vi "BRig_RT_panel_ExpStruct_v1,11.vi"(7 "input_setValues":bool, 11 "input_dataExp":u16[](array[numeric])) -> (3 "output_dataExp":u16[](array[numeric]))   [LabVIEW 2014]
panel:
  in  "I_L_nTrig_PerState":bool
  in  "I_Cue2":bool
  in  "T_Cue2_LED_max":u16=1000 caption="Max" min=5 max=5000 step=5
  in  "T_Cue2_LED_min":u16=1000 caption="Min" min=5 max=5000 step=5
  in  "T_Cue2_LED_step":u16=1000 caption="Penalty" min=1 max=10000 step=1
  in  "T_Cue2_Audio_max":u16=1000 caption="Max" min=5 max=5000 step=5
  in  "T_Cue2_Audio_min":u16=1000 caption="Min" min=5 max=5000 step=5
  in  "T_Cue2_Audio_step":u16=1000 caption="Penalty" min=1 max=10000 step=1
  in  "T_ENL2_step":u16=100 caption="Penalty" min=10 max=10000 step=10
  in  "T_ENL2_max":u16=1000 caption="Max" min=250 max=10000 step=250
  in  "T_ENL2_min":u16=1000 caption="Min" min=250 max=10000 step=250
  in  "ClosedLoop_LaserHold_l2":bool
  in  "ClosedLoop_LaserHold_l1":bool
  in  "FreeReward_Count2":u16
  in  "FreeReward_Count1":u16
  in  "FreeReward_Switch":bool
  in  "T_CuePenalty":u16=1000 caption="Penalty" min=1 max=10000 step=1
  in  "T_ENLPenalty":u16=100 caption="Penalty" min=10 max=10000 step=10
  in  "LaserSwitch_Probability_L1":u16
  in  "LaserSwitch":u16(slide) max=3 step=1 scale=0.0..3.0
  in  "I_allReward":bool caption="NonSpecific\nLick Direction"
  in  "Tcycle_Reward_max_R":u16=1000 caption="Max" min=5 max=5000 step=5
  in  "Tcycle_Reward_min_R":u16=1000 caption="Min" min=5 max=5000 step=5
  in  "Tcycle_Reward_step_R":u16=1000 caption="Penalty" min=1 max=10000 step=1
  in  "Tcycle_Reward_max_L":u16=1000 caption="Max" min=5 max=5000 step=5
  in  "Tcycle_Reward_min_L":u16=1000 caption="Min" min=5 max=5000 step=5
  in  "Tcycle_Reward_step_L":u16=1000 caption="Penalty" min=1 max=10000 step=1
  in  "T_Cue_LED_max":u16=1000 caption="Max" min=5 max=5000 step=5
  in  "T_Cue_LED_min":u16=1000 caption="Min" min=5 max=5000 step=5
  in  "T_Cue_LED_step":u16=1000 caption="Penalty" min=1 max=10000 step=1
  in  "SolenoidProbability_L":u16=100 caption="Reward Time [ms]" min=1 max=1000 step=1
  in  "SolenoidProbability_R":u16=100 caption="Reward Time [ms]" min=1 max=1000 step=1
  in  "T_Cue_Audio_max":u16=1000 caption="Max" min=5 max=5000 step=5
  in  "T_Cue_Audio_min":u16=1000 caption="Min" min=5 max=5000 step=5
  in  "BUR_max":u16 caption="Count Reward Structure  (0 = off)"
  in  "Tcycle_Timeout":u16=1000 caption="Timeout Time [ms]" min=10 max=10000 step=1
  in  "Tcycle_Wrong":u16=1000 caption="Wrong Time [ms]" min=10 max=10000 step=1
  in  "Tcycle_Selection":u16=1000 caption="Answer Time [ms]" min=1 max=10000 step=1
  in  "Tcycle_RewardPost":u16=1000 caption="Consumption Time [ms]" min=250 max=10000 step=250
  in  "TpB_Max_R":u16=4 caption="Max TrialsPerBlock" min=1 max=12 step=1
  in  "TpB_Min_R":u16=4 caption="Min TrialsPerBlock" min=1 max=12 step=1
  in  "TpB_Max_L":u16=4 caption="Max TrialsPerBlock" min=1 max=12 step=1
  in  "TpB_Min_L":u16=4 caption="Min TrialsPerBlock" min=1 max=12 step=1
  in  "BUR_min":u16 caption="Count Reward Structure\n(0 = off)"
  in  "TrialUntilReward":bool caption="Ignore Wrong\nSelection"
  in  "T_Cue_Audio_step":u16=1000 caption="Penalty" min=1 max=10000 step=1
  in  "T_ENL_step":u16=100 caption="Penalty" min=10 max=10000 step=10
  in  "T_ENL_max":u16=1000 caption="Max" min=250 max=10000 step=250
  in  "T_ENL_min":u16=1000 caption="Min" min=250 max=10000 step=250
  # "Experiment Task Structure"
  # "Min            Max               Step        Penalty"
  # "(Laser1 or Laser2)\nLaser1 probability"
  # "Enforced\nNonLick"
  # "Cue Audio"
  # "(ClosedLoop Structure)"
  # "Hold Laser1"
  # "Hold Laser2"
  # "Cue LED"
  # "Allow Multiple Laser\nTriggers During\nENL and Cue?"
  # "Min            Max               Step"
  # "ENL 2"
  # "Cue 2 Audio"
  # "Cue 2 LED"
  # "Selection"
  # "Min"
  # "Max"
  # "Reward - Dispense Water"
  # "Min            Max            StepSize"
  # "Left"
  # "Trial Per Block Structure \n               Left                        Right"
  # "Right"
  # "Min"
  # "Dispense Water Probability"
  # "Max"
  # "%"
  # "Left"
  # "Right"
  # "%"
  # "Give Reward\nIf Too Many Errors"
  # "Reward - Consumption"
  # "# consecutive ReBiasing trials"
  # "Penalty - Wrong Choice"
  # "# consecutive NonForcedError trials"
  # "Penalty - Choice Timeout"
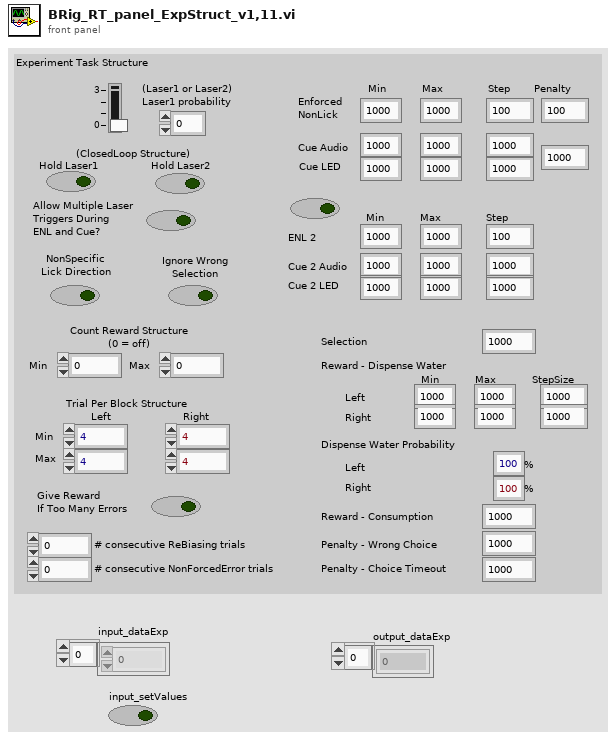
[diagram p1: front panel]
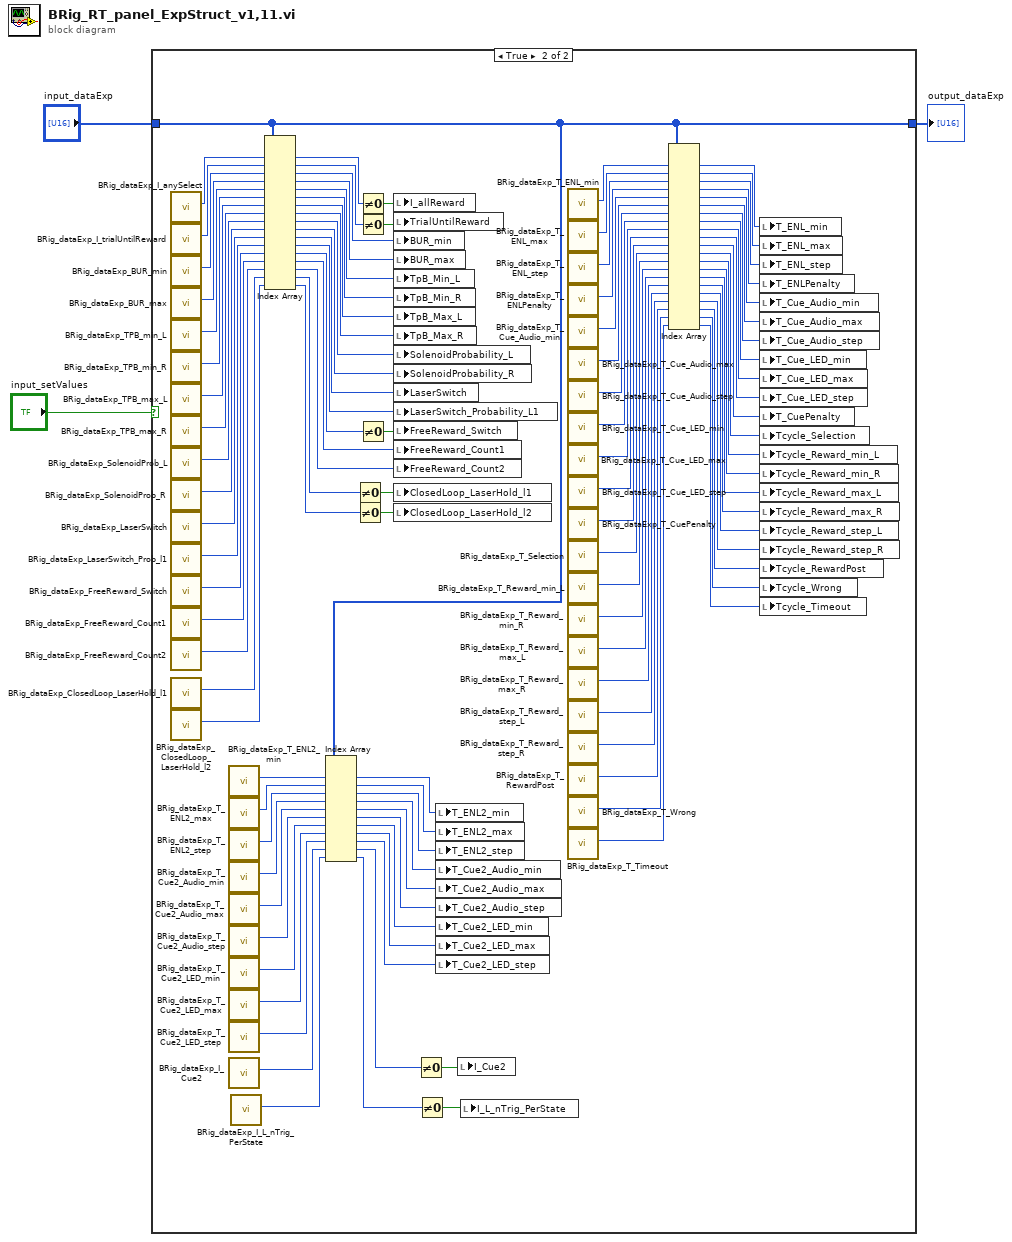
[diagram p0: block diagram]
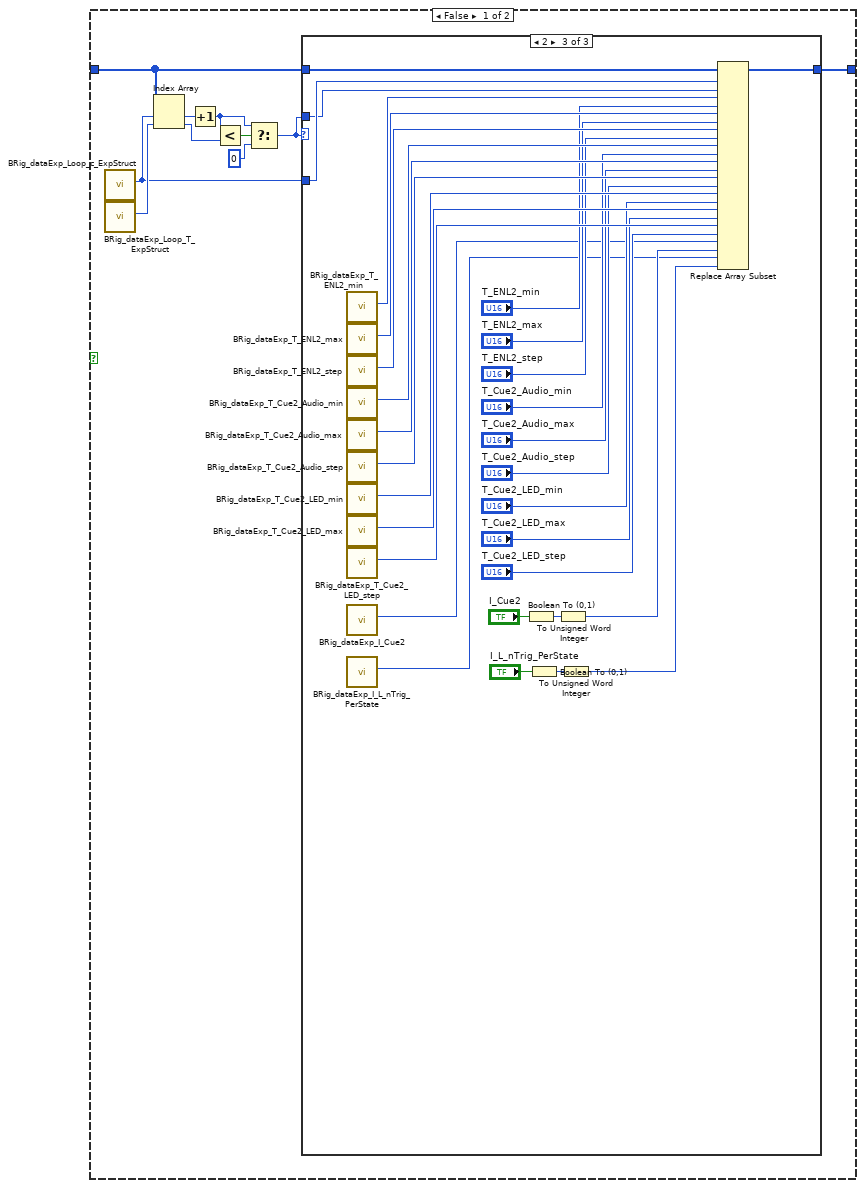
[diagram p2: hidden frame]
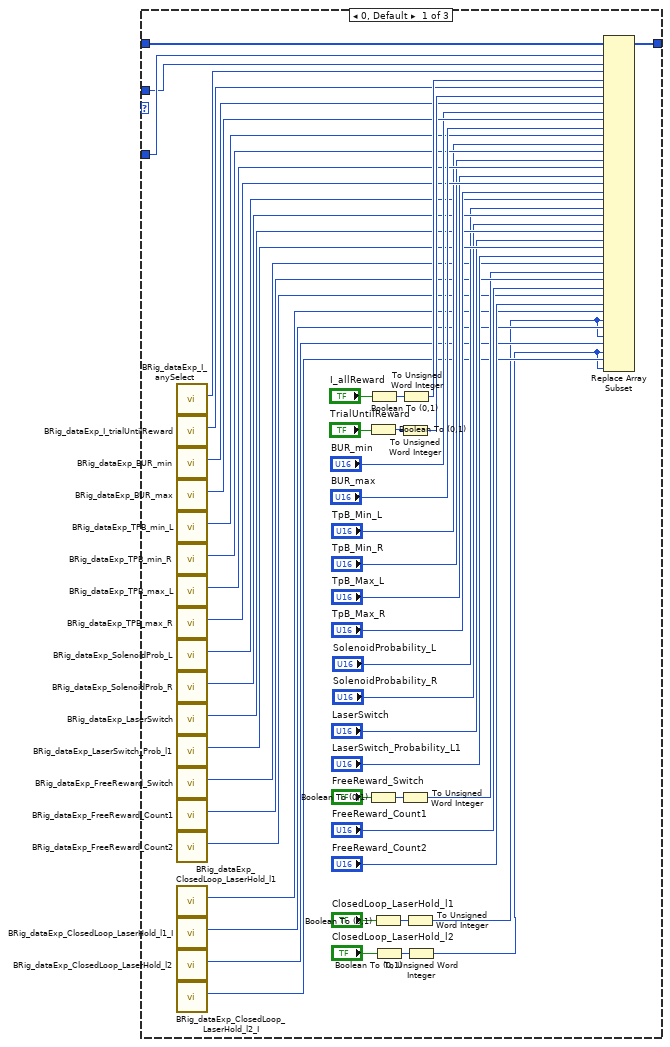
[diagram p3: hidden frame]
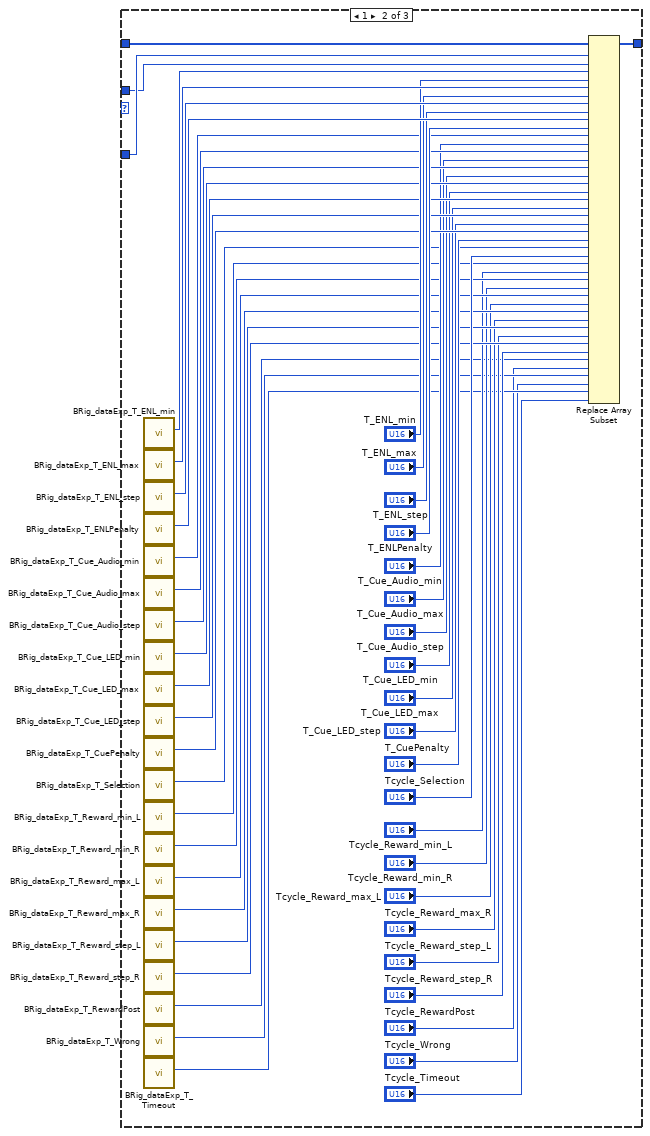
[diagram p4: hidden frame]
diagram:
  n1 = case shown="True" "input_setValues" {
    tunnel: [w13 w164] -> w3
    tunnel: "input_dataExp" -> [w12 w164]
    frame False {
      n2 = call "BRig_dataExp_Loop_c_ExpStruct.vi"() -> ("output_Loop_c_ExpStruct"=w6:i32)  [unwired: 11 in]
      n3 = call "BRig_dataExp_Loop_T_ExpStruct.vi"() -> ("output_Loop_T_ExpStruct"=w11:i32)  [unwired: 11 in]
      n4 = Index Array(array=w12, index #1=w6, index #2=w11) -> (element #1=w10:u16, element #2=w9:u16)
      n5 = Increment(x=w10) -> (x+1=w5:u16)
      n6 = Less?(x=w5, y=w9) -> (x < y?=w8:bool)
      n7 = Select(t=w5, s=w8, f=u16 0) -> (s? t:f=w4:u16)
      n8 = case shown="2" w4 {
        tunnel: w12 -> [w63 w109 w139]
        tunnel: [w62 w108 w138] -> w13
        tunnel: w6 -> [w33 w107 w137]
        tunnel: w4 -> [w32 w106 w136]
        frame 0, Default {
          n9 = call "BRig_dataExp_I_anySelect.vi"() -> ("output_I_anySelect"=w61:i32)  [unwired: 11 in]
          n10 = call "BRig_dataExp_I_trialUntilReward.vi"() -> ("output_I_trialUntilReward"=w57:i32)  [unwired: 11 in]
          n11 = call "BRig_dataExp_BUR_min.vi"() -> ("output_BUR_min"=w53:i32)  [unwired: 11 in]
          n12 = call "BRig_dataExp_BUR_max.vi"() -> ("output_BUR_max"=w52:i32)  [unwired: 11 in]
          n13 = call "BRig_dataExp_TPB_min_L.vi"() -> ("output_TPB_min_L"=w49:i32)  [unwired: 11 in]
          n14 = call "BRig_dataExp_TPB_min_R.vi"() -> ("output_TPB_min_R"=w48:i32)  [unwired: 11 in]
          n15 = call "BRig_dataExp_TPB_max_L.vi"() -> ("output_TPB_max_L"=w47:i32)  [unwired: 11 in]
          n16 = call "BRig_dataExp_TPB_max_R.vi"() -> ("output_TPB_max_R"=w46:i32)  [unwired: 11 in]
          n17 = call "BRig_dataExp_SolenoidProb_L.vi"() -> ("output_SolenoidProbability_L"=w41:i32)  [unwired: 11 in]
          n18 = call "BRig_dataExp_SolenoidProb_R.vi"() -> ("output_SolenoidProbability_R"=w40:i32)  [unwired: 11 in]
          n19 = call "BRig_dataExp_LaserSwitch.vi"() -> ("output_LaserSwitch"=w39:i32)  [unwired: 11 in]
          n20 = call "BRig_dataExp_LaserSwitch_Prob_l1.vi"() -> ("output_LaserSwitch_Probability_L1"=w38:i32)  [unwired: 11 in]
          n21 = call "BRig_dataExp_FreeReward_Switch.vi"() -> ("output_FreeReward_Switch"=w29:i32)  [unwired: 11 in]
          n22 = call "BRig_dataExp_FreeReward_Count1.vi"() -> ("output_FreeReward_Count"=w28:i32)  [unwired: 11 in]
          n23 = call "BRig_dataExp_FreeReward_Count2.vi"() -> ("output_FreeReward_Count"=w25:i32)  [unwired: 11 in]
          n24 = call "BRig_dataExp_ClosedLoop_LaserHold_l1.vi"() -> ("output_CloseLoop_LaserHold_l1"=w23:i32)  [unwired: 11 in]
          n25 = call "BRig_dataExp_ClosedLoop_LaserHold_l1_I.vi"() -> ("output_CloseLoop_LaserHold_l1_I"=w22:i32)  [unwired: 11 in]
          n26 = call "BRig_dataExp_ClosedLoop_LaserHold_l2.vi"() -> ("output_CloseLoop_LaserHold_l2"=w21:i32)  [unwired: 11 in]
          n27 = call "BRig_dataExp_ClosedLoop_LaserHold_l2_I.vi"() -> ("output_CloseLoop_LaserHold_l2_I"=w20:i32)  [unwired: 11 in]
          n28 = Boolean To (0,1)(Boolean="TrialUntilReward") -> (0, 1=w56:i16)
          n29 = Boolean To (0,1)(Boolean="FreeReward_Switch") -> (0, 1=w31:i16)
          n30 = Boolean To (0,1)(Boolean="I_allReward") -> (0, 1=w59:i16)
          n31 = Boolean To (0,1)(Boolean="ClosedLoop_LaserHold_l1") -> (0, 1=w19:i16)
          n32 = Boolean To (0,1)(Boolean="ClosedLoop_LaserHold_l2") -> (0, 1=w17:i16)
          n33 = To Unsigned Word Integer(number=w56) -> (unsigned 16bit integer=w54:u16)
          n34 = To Unsigned Word Integer(number=w31) -> (unsigned 16bit integer=w27:u16)
          n35 = To Unsigned Word Integer(number=w59) -> (unsigned 16bit integer=w58:u16)
          n36 = To Unsigned Word Integer(number=w19) -> (unsigned 16bit integer=w15:u16)
          n37 = To Unsigned Word Integer(number=w17) -> (unsigned 16bit integer=w14:u16)
          n38 = Replace Array Subset(array=w63, new element #1=w32, index #1=w33, new element #2=w58, index #2=w61, new element #3=w54, index #3=w57, new element #4="BUR_min", index #4=w53, new element #5="BUR_max", index #5=w52, new element #6="TpB_Min_L", index #6=w49, new element #7="TpB_Min_R", index #7=w48, new element #8="TpB_Max_L", index #8=w47, new element #9="TpB_Max_R", index #9=w46, new element #10="SolenoidProbability_L", index #10=w41, new element #11="SolenoidProbability_R", index #11=w40, new element #12="LaserSwitch", index #12=w39, new element #13="LaserSwitch_Probability_L1", index #13=w38, new element #14=w27, index #14=w29, new element #15="FreeReward_Count1", index #15=w28, new element #16="FreeReward_Count2", index #16=w25, new element #17=w15, index #17=w23, new element #18=w15, index #18=w22, new element #19=w14, index #19=w21, new element #20=w14, index #20=w20) -> (w62:u16[])
        }
        frame 1 {
          n39 = call "BRig_dataExp_T_ENL_min.vi"() -> ("output_T_ENL_min"=w105:i32)  [unwired: 11 in]
          n40 = call "BRig_dataExp_T_ENL_max.vi"() -> ("output_T_ENL_max"=w104:i32)  [unwired: 11 in]
          n41 = call "BRig_dataExp_T_ENL_step.vi"() -> ("output_T_ENL_step"=w103:i32)  [unwired: 11 in]
          n42 = call "BRig_dataExp_T_ENLPenalty.vi"() -> ("output_ENL_penalty"=w102:i32)  [unwired: 11 in]
          n43 = call "BRig_dataExp_T_Cue_Audio_min.vi"() -> ("output_T_Cue_Audio_min"=w97:i32)  [unwired: 11 in]
          n44 = call "BRig_dataExp_T_Cue_Audio_max.vi"() -> ("output_T_Cue_Audio_max"=w96:i32)  [unwired: 11 in]
          n45 = call "BRig_dataExp_T_Cue_Audio_step.vi"() -> ("output_T_Cue_Audio_step"=w95:i32)  [unwired: 11 in]
          n46 = call "BRig_dataExp_T_Cue_LED_min.vi"() -> ("output_T_Cue_LED_min"=w94:i32)  [unwired: 11 in]
          n47 = call "BRig_dataExp_T_Cue_LED_max.vi"() -> ("output_T_Cue_LED_max"=w93:i32)  [unwired: 11 in]
          n48 = call "BRig_dataExp_T_Cue_LED_step.vi"() -> ("output_T_Cue_LED_step"=w92:i32)  [unwired: 11 in]
          n49 = call "BRig_dataExp_T_CuePenalty.vi"() -> ("output_T_CuePenalty"=w91:i32)  [unwired: 11 in]
          n50 = call "BRig_dataExp_T_Selection.vi"() -> ("output_T_Selection"=w83:i32)  [unwired: 11 in]
          n51 = call "BRig_dataExp_T_Reward_min_L.vi"() -> ("output_Tcycle_Reward_min_L"=w81:i32)  [unwired: 11 in]
          n52 = call "BRig_dataExp_T_Reward_min_R.vi"() -> ("output_T_Reward_min_R"=w80:i32)  [unwired: 11 in]
          n53 = call "BRig_dataExp_T_Reward_max_L.vi"() -> ("output_T_Reward_max_L"=w79:i32)  [unwired: 11 in]
          n54 = call "BRig_dataExp_T_Reward_max_R.vi"() -> ("output_T_Reward_max_R"=w78:i32)  [unwired: 11 in]
          n55 = call "BRig_dataExp_T_Reward_step_L.vi"() -> ("output_T_Reward_step_L"=w77:i32)  [unwired: 11 in]
          n56 = call "BRig_dataExp_T_Reward_step_R.vi"() -> ("output_T_Reward_step_R"=w76:i32)  [unwired: 11 in]
          n57 = call "BRig_dataExp_T_RewardPost.vi"() -> ("output_T_RewardPost"=w69:i32)  [unwired: 11 in]
          n58 = call "BRig_dataExp_T_Wrong.vi"() -> ("output_T_Wrong"=w68:i32)  [unwired: 11 in]
          n59 = call "BRig_dataExp_T_Timeout.vi"() -> ("output_T_Timeout"=w67:i32)  [unwired: 11 in]
          n60 = Replace Array Subset(array=w109, new element #1=w106, index #1=w107, new element #2="T_ENL_min", index #2=w105, new element #3="T_ENL_max", index #3=w104, new element #4="T_ENL_step", index #4=w103, new element #5="T_ENLPenalty", index #5=w102, new element #6="T_Cue_Audio_min", index #6=w97, new element #7="T_Cue_Audio_max", index #7=w96, new element #8="T_Cue_Audio_step", index #8=w95, new element #9="T_Cue_LED_min", index #9=w94, new element #10="T_Cue_LED_max", index #10=w93, new element #11="T_Cue_LED_step", index #11=w92, new element #12="T_CuePenalty", index #12=w91, new element #13="Tcycle_Selection", index #13=w83, new element #14="Tcycle_Reward_min_L", index #14=w81, new element #15="Tcycle_Reward_min_R", index #15=w80, new element #16="Tcycle_Reward_max_L", index #16=w79, new element #17="Tcycle_Reward_max_R", index #17=w78, new element #18="Tcycle_Reward_step_L", index #18=w77, new element #19="Tcycle_Reward_step_R", index #19=w76, new element #20="Tcycle_RewardPost", index #20=w69, new element #21="Tcycle_Wrong", index #21=w68, new element #22="Tcycle_Timeout", index #22=w67) -> (w108:u16[])
        }
        frame 2 {
          n61 = call "BRig_dataExp_T_ENL2_min.vi"() -> ("output_T_ENL2_min"=w135:i32)  [unwired: 11 in]
          n62 = call "BRig_dataExp_T_ENL2_max.vi"() -> ("output_T_ENL2_max"=w134:i32)  [unwired: 11 in]
          n63 = call "BRig_dataExp_T_ENL2_step.vi"() -> ("output_T_ENL2_step"=w133:i32)  [unwired: 11 in]
          n64 = call "BRig_dataExp_T_Cue2_Audio_min.vi"() -> ("output_T_Cue2_Audio_min"=w132:i32)  [unwired: 11 in]
          n65 = call "BRig_dataExp_T_Cue2_Audio_max.vi"() -> ("output_T_Cue2_Audio_max"=w131:i32)  [unwired: 11 in]
          n66 = call "BRig_dataExp_T_Cue2_Audio_step.vi"() -> ("output_T_Cue2_Audio_step"=w130:i32)  [unwired: 11 in]
          n67 = call "BRig_dataExp_T_Cue2_LED_min.vi"() -> ("output_T_Cue2_LED_min"=w129:i32)  [unwired: 11 in]
          n68 = call "BRig_dataExp_T_Cue2_LED_max.vi"() -> ("output_T_Cue2_LED_max"=w128:i32)  [unwired: 11 in]
          n69 = call "BRig_dataExp_T_Cue2_LED_step.vi"() -> ("output_T_Cue2_LED_step"=w127:i32)  [unwired: 11 in]
          n70 = call "BRig_dataExp_I_Cue2.vi"() -> ("output_I_Cue2"=w117:i32)  [unwired: 11 in]
          n71 = call "BRig_dataExp_I_L_nTrig_PerState.vi"() -> ("output_I_L_nTrig_PerState"=w113:i32)  [unwired: 11 in]
          n72 = Boolean To (0,1)(Boolean="I_Cue2") -> (0, 1=w115:i16)
          n73 = Boolean To (0,1)(Boolean="I_L_nTrig_PerState") -> (0, 1=w112:i16)
          n74 = To Unsigned Word Integer(number=w115) -> (unsigned 16bit integer=w114:u16)
          n75 = To Unsigned Word Integer(number=w112) -> (unsigned 16bit integer=w110:u16)
          n76 = Replace Array Subset(array=w139, new element #1=w136, index #1=w137, new element #2="T_ENL2_min", index #2=w135, new element #3="T_ENL2_max", index #3=w134, new element #4="T_ENL2_step", index #4=w133, new element #5="T_Cue2_Audio_min", index #5=w132, new element #6="T_Cue2_Audio_max", index #6=w131, new element #7="T_Cue2_Audio_step", index #7=w130, new element #8="T_Cue2_LED_min", index #8=w129, new element #9="T_Cue2_LED_max", index #9=w128, new element #10="T_Cue2_LED_step", index #10=w127, new element #11=w114, index #11=w117, new element #12=w110, index #12=w113) -> (w138:u16[])
        }
      }
    }
    frame True {
      n77 = call "BRig_dataExp_I_anySelect.vi"() -> ("output_I_anySelect"=w245:i32)  [unwired: 11 in]
      n78 = call "BRig_dataExp_I_trialUntilReward.vi"() -> ("output_I_trialUntilReward"=w244:i32)  [unwired: 11 in]
      n79 = call "BRig_dataExp_BUR_min.vi"() -> ("output_BUR_min"=w243:i32)  [unwired: 11 in]
      n80 = call "BRig_dataExp_BUR_max.vi"() -> ("output_BUR_max"=w242:i32)  [unwired: 11 in]
      n81 = call "BRig_dataExp_TPB_min_L.vi"() -> ("output_TPB_min_L"=w241:i32)  [unwired: 11 in]
      n82 = call "BRig_dataExp_TPB_min_R.vi"() -> ("output_TPB_min_R"=w240:i32)  [unwired: 11 in]
      n83 = call "BRig_dataExp_TPB_max_L.vi"() -> ("output_TPB_max_L"=w239:i32)  [unwired: 11 in]
      n84 = call "BRig_dataExp_TPB_max_R.vi"() -> ("output_TPB_max_R"=w238:i32)  [unwired: 11 in]
      n85 = call "BRig_dataExp_SolenoidProb_L.vi"() -> ("output_SolenoidProbability_L"=w237:i32)  [unwired: 11 in]
      n86 = call "BRig_dataExp_SolenoidProb_R.vi"() -> ("output_SolenoidProbability_R"=w236:i32)  [unwired: 11 in]
      n87 = call "BRig_dataExp_LaserSwitch.vi"() -> ("output_LaserSwitch"=w235:i32)  [unwired: 11 in]
      n88 = call "BRig_dataExp_LaserSwitch_Prob_l1.vi"() -> ("output_LaserSwitch_Probability_L1"=w234:i32)  [unwired: 11 in]
      n89 = call "BRig_dataExp_FreeReward_Switch.vi"() -> ("output_FreeReward_Switch"=w233:i32)  [unwired: 11 in]
      n90 = call "BRig_dataExp_FreeReward_Count1.vi"() -> ("output_FreeReward_Count"=w232:i32)  [unwired: 11 in]
      n91 = call "BRig_dataExp_FreeReward_Count2.vi"() -> ("output_FreeReward_Count"=w172:i32)  [unwired: 11 in]
      n92 = call "BRig_dataExp_ClosedLoop_LaserHold_l1.vi"() -> ("output_CloseLoop_LaserHold_l1"=w170:i32)  [unwired: 11 in]
      n93 = call "BRig_dataExp_ClosedLoop_LaserHold_l2.vi"() -> ("output_CloseLoop_LaserHold_l2"=w169:i32)  [unwired: 11 in]
      n94 = call "BRig_dataExp_T_ENL2_min.vi"() -> ("output_T_ENL2_min"=w163:i32)  [unwired: 11 in]
      n95 = call "BRig_dataExp_T_ENL2_max.vi"() -> ("output_T_ENL2_max"=w162:i32)  [unwired: 11 in]
      n96 = call "BRig_dataExp_T_ENL2_step.vi"() -> ("output_T_ENL2_step"=w161:i32)  [unwired: 11 in]
      n97 = call "BRig_dataExp_T_Cue2_Audio_min.vi"() -> ("output_T_Cue2_Audio_min"=w160:i32)  [unwired: 11 in]
      n98 = call "BRig_dataExp_T_Cue2_Audio_max.vi"() -> ("output_T_Cue2_Audio_max"=w159:i32)  [unwired: 11 in]
      n99 = call "BRig_dataExp_T_Cue2_Audio_step.vi"() -> ("output_T_Cue2_Audio_step"=w158:i32)  [unwired: 11 in]
      n100 = call "BRig_dataExp_T_Cue2_LED_min.vi"() -> ("output_T_Cue2_LED_min"=w157:i32)  [unwired: 11 in]
      n101 = call "BRig_dataExp_T_Cue2_LED_max.vi"() -> ("output_T_Cue2_LED_max"=w156:i32)  [unwired: 11 in]
      n102 = call "BRig_dataExp_T_Cue2_LED_step.vi"() -> ("output_T_Cue2_LED_step"=w155:i32)  [unwired: 11 in]
      n103 = call "BRig_dataExp_I_Cue2.vi"() -> ("output_I_Cue2"=w145:i32)  [unwired: 11 in]
      n104 = call "BRig_dataExp_I_L_nTrig_PerState.vi"() -> ("output_I_L_nTrig_PerState"=w142:i32)  [unwired: 11 in]
      n105 = Index Array(array=w164, index #1=w245, index #2=w244, index #3=w243, index #4=w242, index #5=w241, index #6=w240, index #7=w239, index #8=w238, index #9=w237, index #10=w236, index #11=w235, index #12=w234, index #13=w233, index #14=w232, index #15=w172, index #16=w170, index #17=w169) -> (element #1=w228:u16, element #2=w227:u16, element #3=w226:u16, element #4=w225:u16, element #5=w224:u16, element #6=w223:u16, element #7=w222:u16, element #8=w221:u16, element #9=w220:u16, element #10=w219:u16, element #11=w218:u16, element #12=w217:u16, element #13=w216:u16, element #14=w215:u16, element #15=w171:u16, element #16=w166:u16, element #17=w165:u16)
      n106 = Index Array(array=w164, index #1=w163, index #2=w162, index #3=w161, index #4=w160, index #5=w159, index #6=w158, index #7=w157, index #8=w156, index #9=w155, index #10=w145, index #11=w142) -> (element #1=w154:u16, element #2=w153:u16, element #3=w152:u16, element #4=w151:u16, element #5=w150:u16, element #6=w149:u16, element #7=w148:u16, element #8=w147:u16, element #9=w146:u16, element #10=w143:u16, element #11=w141:u16)
      n107 = Not Equal To 0?(x=w166) -> (x != 0?=w168:bool)
      n108 = Not Equal To 0?(x=w165) -> (x != 0?=w167:bool)
      n109 = Not Equal To 0?(x=w228) -> (x != 0?=w231:bool)
      n110 = Not Equal To 0?(x=w227) -> (x != 0?=w230:bool)
      n111 = Not Equal To 0?(x=w216) -> (x != 0?=w229:bool)
      n112 = local write "I_allReward"(w231) -> ()
      n113 = local write "TrialUntilReward"(w230) -> ()
      n114 = local write "BUR_min"(w226) -> ()
      n115 = local write "BUR_max"(w225) -> ()
      n116 = local write "TpB_Min_L"(w224) -> ()
      n117 = local write "TpB_Min_R"(w223) -> ()
      n118 = local write "TpB_Max_L"(w222) -> ()
      n119 = local write "TpB_Max_R"(w221) -> ()
      n120 = local write "SolenoidProbability_L"(w220) -> ()
      n121 = local write "SolenoidProbability_R"(w219) -> ()
      n122 = local write "LaserSwitch"(w218) -> ()
      n123 = local write "LaserSwitch_Probability_L1"(w217) -> ()
      n124 = local write "FreeReward_Switch"(w229) -> ()
      n125 = local write "FreeReward_Count1"(w215) -> ()
      n126 = local write "FreeReward_Count2"(w171) -> ()
      n127 = local write "ClosedLoop_LaserHold_l1"(w168) -> ()
      n128 = local write "ClosedLoop_LaserHold_l2"(w167) -> ()
      n129 = Not Equal To 0?(x=w143) -> (x != 0?=w144:bool)
      n130 = Not Equal To 0?(x=w141) -> (x != 0?=w140:bool)
      n131 = local write "T_ENL2_min"(w154) -> ()
      n132 = local write "T_ENL2_max"(w153) -> ()
      n133 = local write "T_ENL2_step"(w152) -> ()
      n134 = local write "T_Cue2_Audio_min"(w151) -> ()
      n135 = local write "T_Cue2_Audio_max"(w150) -> ()
      n136 = local write "T_Cue2_Audio_step"(w149) -> ()
      n137 = local write "T_Cue2_LED_min"(w148) -> ()
      n138 = local write "T_Cue2_LED_max"(w147) -> ()
      n139 = local write "T_Cue2_LED_step"(w146) -> ()
      n140 = local write "I_Cue2"(w144) -> ()
      n141 = local write "I_L_nTrig_PerState"(w140) -> ()
      n142 = call "BRig_dataExp_T_ENL_min.vi"() -> ("output_T_ENL_min"=w214:i32)  [unwired: 11 in]
      n143 = call "BRig_dataExp_T_ENL_max.vi"() -> ("output_T_ENL_max"=w213:i32)  [unwired: 11 in]
      n144 = call "BRig_dataExp_T_ENL_step.vi"() -> ("output_T_ENL_step"=w212:i32)  [unwired: 11 in]
      n145 = call "BRig_dataExp_T_ENLPenalty.vi"() -> ("output_ENL_penalty"=w211:i32)  [unwired: 11 in]
      n146 = call "BRig_dataExp_T_Cue_Audio_min.vi"() -> ("output_T_Cue_Audio_min"=w210:i32)  [unwired: 11 in]
      n147 = call "BRig_dataExp_T_Cue_Audio_max.vi"() -> ("output_T_Cue_Audio_max"=w209:i32)  [unwired: 11 in]
      n148 = call "BRig_dataExp_T_Cue_Audio_step.vi"() -> ("output_T_Cue_Audio_step"=w208:i32)  [unwired: 11 in]
      n149 = call "BRig_dataExp_T_Cue_LED_min.vi"() -> ("output_T_Cue_LED_min"=w207:i32)  [unwired: 11 in]
      n150 = call "BRig_dataExp_T_Cue_LED_max.vi"() -> ("output_T_Cue_LED_max"=w206:i32)  [unwired: 11 in]
      n151 = call "BRig_dataExp_T_Cue_LED_step.vi"() -> ("output_T_Cue_LED_step"=w205:i32)  [unwired: 11 in]
      n152 = call "BRig_dataExp_T_CuePenalty.vi"() -> ("output_T_CuePenalty"=w204:i32)  [unwired: 11 in]
      n153 = call "BRig_dataExp_T_Selection.vi"() -> ("output_T_Selection"=w203:i32)  [unwired: 11 in]
      n154 = call "BRig_dataExp_T_Reward_min_L.vi"() -> ("output_Tcycle_Reward_min_L"=w202:i32)  [unwired: 11 in]
      n155 = call "BRig_dataExp_T_Reward_min_R.vi"() -> ("output_T_Reward_min_R"=w201:i32)  [unwired: 11 in]
      n156 = call "BRig_dataExp_T_Reward_max_L.vi"() -> ("output_T_Reward_max_L"=w200:i32)  [unwired: 11 in]
      n157 = call "BRig_dataExp_T_Reward_max_R.vi"() -> ("output_T_Reward_max_R"=w199:i32)  [unwired: 11 in]
      n158 = call "BRig_dataExp_T_Reward_step_L.vi"() -> ("output_T_Reward_step_L"=w198:i32)  [unwired: 11 in]
      n159 = call "BRig_dataExp_T_Reward_step_R.vi"() -> ("output_T_Reward_step_R"=w197:i32)  [unwired: 11 in]
      n160 = call "BRig_dataExp_T_RewardPost.vi"() -> ("output_T_RewardPost"=w196:i32)  [unwired: 11 in]
      n161 = call "BRig_dataExp_T_Wrong.vi"() -> ("output_T_Wrong"=w195:i32)  [unwired: 11 in]
      n162 = call "BRig_dataExp_T_Timeout.vi"() -> ("output_T_Timeout"=w194:i32)  [unwired: 11 in]
      n163 = Index Array(array=w164, index #1=w214, index #2=w213, index #3=w212, index #4=w211, index #5=w210, index #6=w209, index #7=w208, index #8=w207, index #9=w206, index #10=w205, index #11=w204, index #12=w203, index #13=w202, index #14=w201, index #15=w200, index #16=w199, index #17=w198, index #18=w197, index #19=w196, index #20=w195, index #21=w194) -> (element #1=w193:u16, element #2=w192:u16, element #3=w191:u16, element #4=w190:u16, element #5=w189:u16, element #6=w188:u16, element #7=w187:u16, element #8=w186:u16, element #9=w185:u16, element #10=w184:u16, element #11=w183:u16, element #12=w182:u16, element #13=w181:u16, element #14=w180:u16, element #15=w179:u16, element #16=w178:u16, element #17=w177:u16, element #18=w176:u16, element #19=w175:u16, element #20=w174:u16, element #21=w173:u16)
      n164 = local write "T_ENL_min"(w193) -> ()
      n165 = local write "T_ENL_max"(w192) -> ()
      n166 = local write "T_ENL_step"(w191) -> ()
      n167 = local write "T_ENLPenalty"(w190) -> ()
      n168 = local write "T_Cue_Audio_min"(w189) -> ()
      n169 = local write "T_Cue_Audio_max"(w188) -> ()
      n170 = local write "T_Cue_Audio_step"(w187) -> ()
      n171 = local write "T_Cue_LED_min"(w186) -> ()
      n172 = local write "T_Cue_LED_max"(w185) -> ()
      n173 = local write "T_Cue_LED_step"(w184) -> ()
      n174 = local write "T_CuePenalty"(w183) -> ()
      n175 = local write "Tcycle_Selection"(w182) -> ()
      n176 = local write "Tcycle_Reward_min_L"(w181) -> ()
      n177 = local write "Tcycle_Reward_min_R"(w180) -> ()
      n178 = local write "Tcycle_Reward_max_L"(w179) -> ()
      n179 = local write "Tcycle_Reward_max_R"(w178) -> ()
      n180 = local write "Tcycle_Reward_step_L"(w177) -> ()
      n181 = local write "Tcycle_Reward_step_R"(w176) -> ()
      n182 = local write "Tcycle_RewardPost"(w175) -> ()
      n183 = local write "Tcycle_Wrong"(w174) -> ()
      n184 = local write "Tcycle_Timeout"(w173) -> ()
    }
  }
  "output_dataExp" <- w3
